vi "jaccard kNN.vi"() -> ()   [LabVIEW 2014]
uses:
  <vilib>/Utility/file.llb/Write To Spreadsheet File (string).vi
panel:
  out "Array 4":string[][](array[string])
  out "Slide 2":dbl(slide) scale=0.0..50.0
  out "Slide":dbl(slide) scale=0.0..9.0
  in  "Path":path
  in  "all rows":string[][](array[string])=array2038x3[6114 elements]
  out "LCS/min (Lsample,Lknown)":dbl[][](array[numeric])
  out "Distance values (LCS)":dbl[][](array[numeric])
  out "size(s)":i32
  out "accuracy":string[][](array[string])
  out "Results":string[][](array[string])
  out "test data (K)":string[][](array[string])
  out "training data (k-1)":string[][](array[string])
  in  "K folds K":i32=10
  out "K folds data":string[][](array[string])
  out "Assigned using LCS (enhanced)":string[][](array[string])
  out "Assigned using LCS":string[][](array[string])
  in  "class labels for training data":string[](array[string])
  in  "kNN k":i32=5
  in  "training data (cluster centers)":string[](array[string])
  in  "test data (patterns in)":string[](array[string])=["0 4 0", "4 0 4", "0 4 0", "4 0 4", "0 4 0", "4 0 4", "0 4 0", "4 0 -2", "0 -2 3", "-2 3 0", "3 0 3", "0 3 0", "3 0 4", "0 4 0", "-2 0 1", "0 1 0", "1 0 -4", "0 -4 4", "-2 2 0", "2 0 -1", "0 -1 -4", "-1 -4 1", "-4 1 0", "1 0 3", "0 3 0", "-1 0 -1", "0 -1 2", "0 -1 1", "-1 1 0", "1 0 4", "0 4 0", "4 0 3", "0 3 -2", "3 -2 0", "-2 0 -2", "0 -2 3", "-2 3 -2", "3 -2 0", "-2 0 4", "0 4 0", "4 0 -2", "0 -2 2", "2 -1 0", "-1 0 4", "0 4 0", "4 0 2", "0 2 0", "2 0 -2", "0 -2 0", "1 -1 0", "-1 0 3", "0 3 0", "3 0 -4", "0 -4 4", "-4 4 -4", "4 -4 0", "2 -1 0", "-1 0 3", "0 3 -2", "3 -2 0", "-2 0 -3", "0 -3 0", "-3 0 3", "0 3 0", "3 0 -3", "0 -3 0", "0 4 0", "4 0 4", "0 4 -4", "4 -4 1", "-4 1 -1", "1 -1 0", "-1 0 -3", "0 -3 0", "-3 0 1", "0 1 -4", "1 -4 1", "-4 1 0", "1 0 4", "0 4 0", "4 0 -4", "0 -4 0", "-4 0 -4", "0 -4 4", "-4 4 -4", "4 -4 1", "0 -4 1", "-4 1 0", "1 0 -4", "0 -4 4", "0 4 0", "4 0 -2", "0 -2 2", "-2 2 -2", "2 -2 2", "-2 2 -2", "2 -2 2", "-2 2 -1", "2 -1 0", "-1 0 4", "0 4 0", "4 0 2", "0 2 0", "2 0 4", "0 4 0", "4 0 2", "0 2 -2", "2 -2 0", "-2 0 4", "1 0 -1", "0 -1 0", "-1 0 -1", "0 -1 0", "-1 0 1", "0 1 -1", "-2 2 -2", "2 -2 3", "1 0 -1", "0 -1 0", "-1 0 -1", "0 -1 2", "-1 2 0", "2 0 2", "0 2 -2", "2 -2 0", "-2 0 -4", "0 -4 0", "-2 2 0", "2 0 3", "0 3 -2", "3 -2 2", "1 -1 0", "-1 0 3", "0 4 0", "-2 0 1", "0 1 -4", "1 -4 0", "-4 0 -3", "0 -3 0", "1 0 -1", "0 -1 2", "-1 2 -1", "2 -1 1", "-1 1 -4", "-2 0 -1", "0 -1 1", "0 3 0", "3 0 3", "0 3 0", "3 0 3", "0 3 -2", "-4 0 -4", "0 -4 4", "0 4 0", "4 0 -4", "0 -4 0", "-4 0 -4", "-2 2 0", "2 0 4", "0 4 -4", "4 -4 0", "-4 0 2", "0 2 -2"]
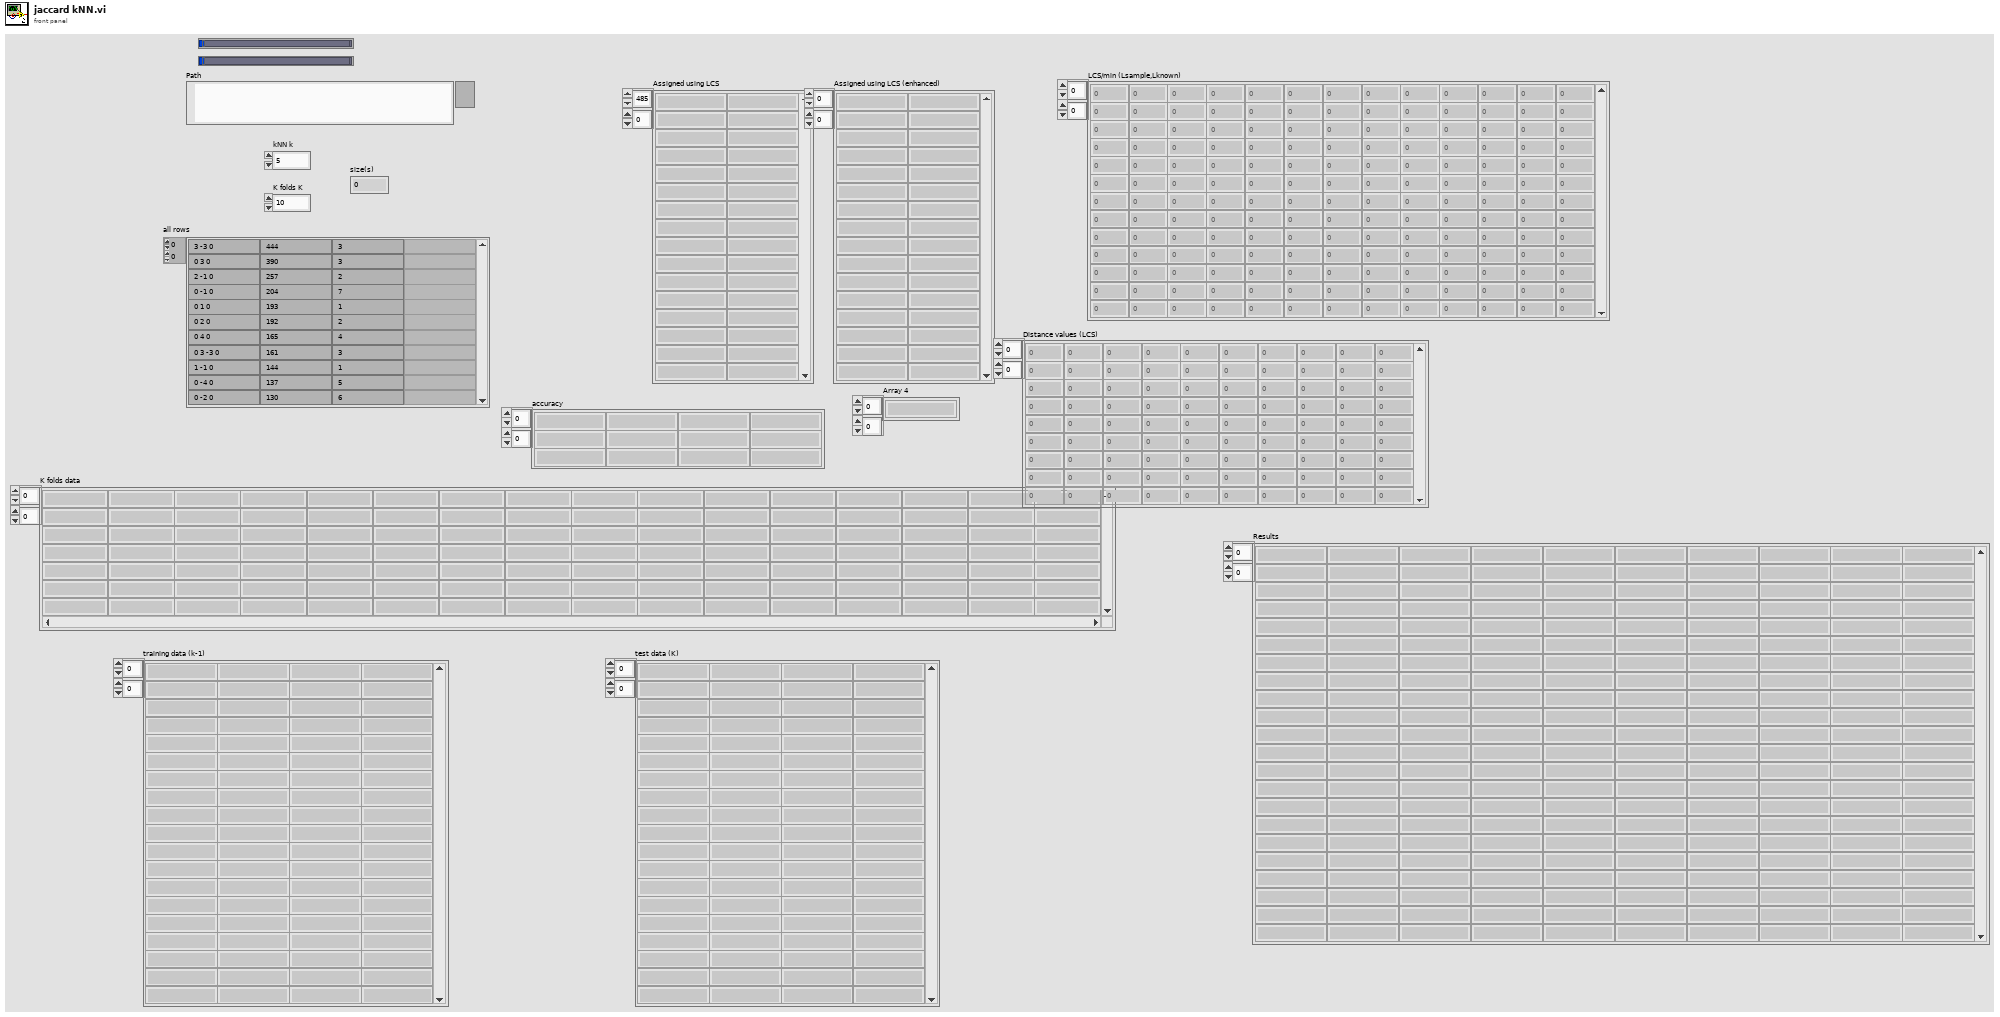
[diagram p1: front panel]
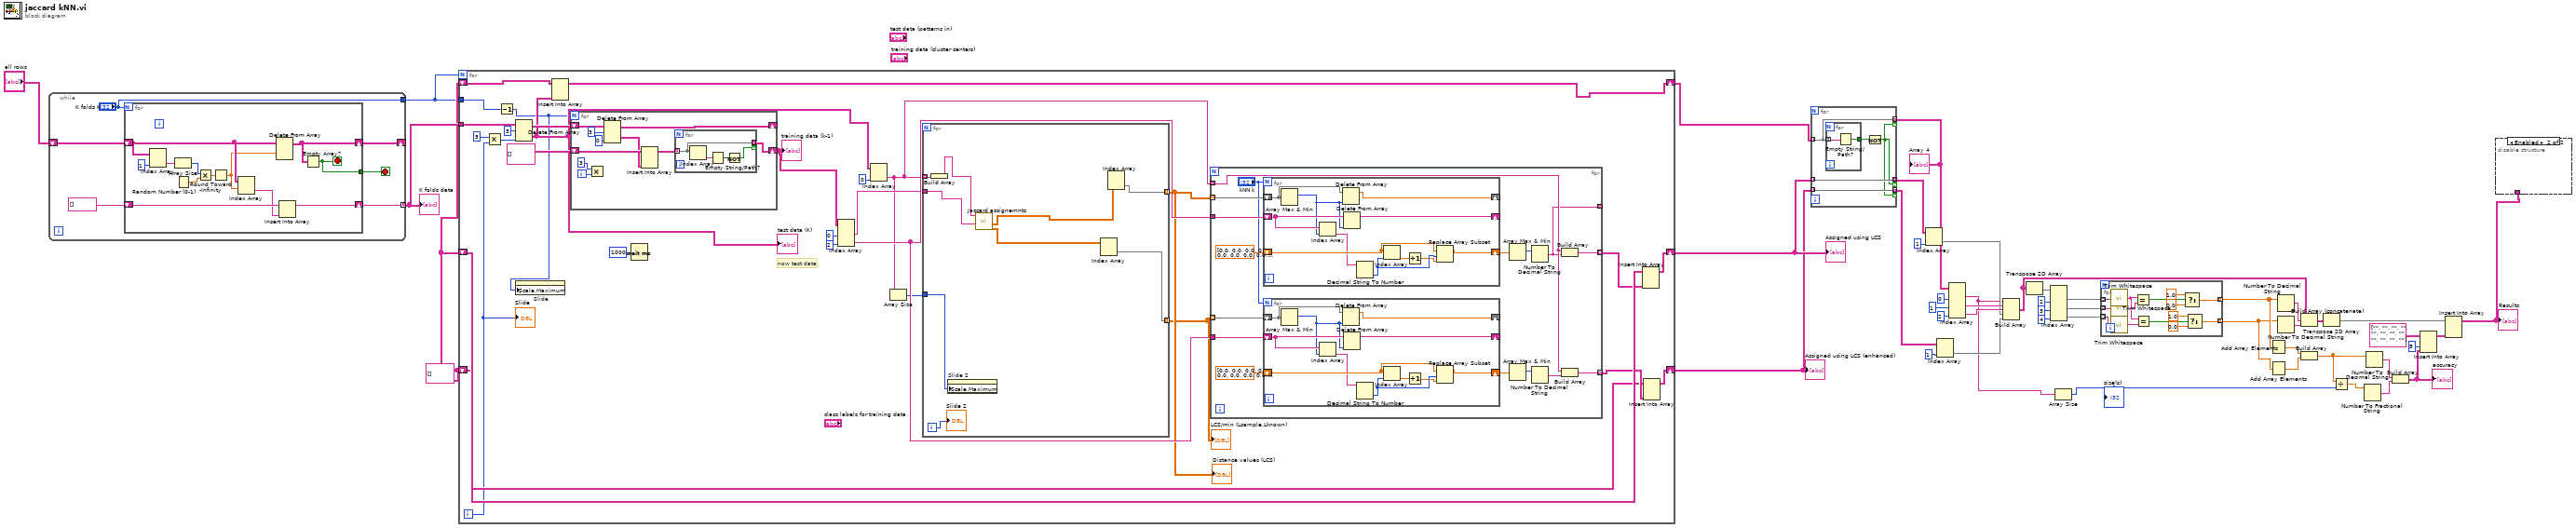
[diagram p0: block diagram]
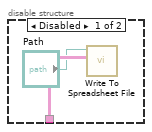
[diagram p2: hidden frame]
diagram:
  w10 = string[][] []
  n1 = while {
    shift-right: [w49] -> _
    shift-left: "all rows" -> [w50]
    tunnel: [w51] -> w46 mode=indexing
    tunnel: ["K folds K"] -> w2
    stop <- w48 stop-if-true
    n2 = for {
      N: "K folds K" -> [_]
      shift-right: [w57] -> w51
      shift-left: string[] [] ("all rows 2") -> [w64]
      shift-right: [w55] -> w49
      shift-left: w50 -> [w56]
      tunnel: [w54] -> w48
      stop <- w54 stop-if-true
      n3 = Index Array(array=w56, index (col)=1 ("disabled index (col)")) -> (element=w60:string[])  [unwired: 1 in]
      n4 = Array Size(array=w60) -> (size(s)=w61:i32)
      n5 = Random Number (0-1)() -> (number: 0 to 1=w62:dbl)
      n6 = Multiply(x=w61, y=w62) -> (x*y=w63:dbl)
      n7 = Round Toward -Infinity(1:w63) -> (0:w53:dbl)
      n8 = Index Array(array=w56, index (row)=w53) -> (element=w58:string[])  [unwired: 1 in]
      n9 = Delete From Array(array=w56, index (row)=w53) -> (array with subset deleted=w55:string[][])  [unwired: 2 in, 1 out]
      n10 = Insert Into Array(array=w64, new element=w58) -> (w57:string[])  [unwired: 1 in]
      n11 = Empty Array?(array=w55) -> (empty?=w54:bool)
    }
  }
  "K folds data" <- w46
  n12 = for {
    N: w2 -> [_]
    tunnel: w46 -> [w93]
    tunnel: w2 -> [w69]
    shift-right: [w76] -> w8
    shift-left: w10 -> [w78]
    shift-right: [w73] -> w7
    shift-left: w10 -> [w75]
    shift-right: [w70] -> w5
    shift-left: w10 -> [w71]
    i -> [w68]
    # "now test data"
    n13 = Multiply(x=3, y=w68) -> (x*y=w82:i32)
    n14 = Decrement(x=w69) -> (x-1=w65:i32)
    n15 = Delete From Array(array=w93, length=3, index (col)=w82) -> (deleted portion=w77:string[][], array with subset deleted=w81:string[][])  [unwired: 1 in]
    "test data (K)" <- w77
    n16 = property on="Slide" class="Slide (strict)"("Scale.Maximum"=w65) -> ()  [unwired: 2 in, 2 out]
    n17 = Insert Into Array(array=w78, new element=w77) -> (w76:string[][])  [unwired: 2 in]
    n18 = for {
      N: w65 -> [_]
      shift-right: [w94] -> w85
      shift-left: string[][] [] ("all rows 2") -> [w102]
      shift-right: [w97] -> _
      shift-left: w81 -> [w103]
      i -> [w99]
      n19 = Multiply(x=3, y=w99) -> ()  [unwired: 1 out]
      n20 = Delete From Array(array=w103, length=3 ("index (col)"), index (col)=0 ("disabled index (col)")) -> (deleted portion=w101:string[][], array with subset deleted=w97:string[][])  [unwired: 1 in]
      n21 = Insert Into Array(array=w102, new element=w101) -> (w95:string[][])  [unwired: 2 in]
      n22 = for {
        tunnel: w95 -> [w106] mode=indexing
        tunnel: [w106] -> w94 mode=indexing if=w107
        n23 = Index Array(array=w106) -> (element=w105:string)  [unwired: 1 in]
        n24 = Empty String/Path?(string/path=w105) -> (empty?=w104:bool)
        n25 = Not(x=w104) -> (.not. x?=w107:bool)
      }
    }
    "training data (k-1)" <- w85
    n26 = Wait (ms)(milliseconds to wait=u32 1000) -> ()  [unwired: 1 out]
    n27 = Index Array(array=w85, index (col) #1=0 ("disabled index (col)"), index (col) #2=2 ("index (col)")) -> (element #1=w88:string[], element #2=w89:string[])  [unwired: 2 in]
    n28 = Index Array(array=w77, index (col)=0 ("disabled index (col)")) -> (element=w67:string[])  [unwired: 1 in]
    n29 = Array Size(array=w67) -> (size(s)=w66:i32)
    n30 = for {
      tunnel: w67 -> [w154] mode=indexing
      tunnel: w88 -> [w150]
      tunnel: [w149] -> w87 mode=indexing
      tunnel: [w148] -> w86 mode=indexing
      tunnel: w66 -> [w152]
      i -> [w153]
      n31 = Build Array(w154) -> (w151:string[])
      n32 = property on="Slide 2" class="Slide (strict)"("Scale.Maximum"=w152) -> ()  [unwired: 2 in, 2 out]
      n33 = call "Jaccard assignemnts.vi"("cluster centers in"=w150, "patterns in"=w151) -> ("distance values out enhanced multiset)"=w147:dbl[][], "distance values out (multiset)"=w146:dbl[][])  [unwired: 6 in, 2 out]
      n34 = Index Array(array=w147) -> (element=w148:dbl[])  [unwired: 2 in]
      n35 = Index Array(array=w146) -> (element=w149:dbl[])  [unwired: 2 in]
      "Slide 2" <- w153
    }
    "Distance values (LCS)" <- w87
    "LCS/min (Lsample,Lknown)" <- w86
    n36 = for {
      tunnel: w67 -> [w114] mode=indexing
      tunnel: w87 -> [w123] mode=indexing
      tunnel: w89 -> [w122]
      tunnel: w86 -> [w113] mode=indexing
      tunnel: w89 -> [w112]
      tunnel: [w111] -> w74 mode=indexing
      tunnel: [w110] -> w72 mode=indexing
      tunnel: [w108] -> _ mode=indexing
      n37 = for {
        N: "kNN k" -> [_]
        shift-right: [w142] -> _
        shift-left: w123 -> [w145]
        shift-right: [w141] -> _
        shift-left: w122 -> [w144]
        shift-right: [w136] -> w119
        shift-left: dbl[] [0.0, 0.0, 0.0, 0.0, 0.0, 0.0, 0.0, 0.0, 0.0, 0.0, 0.0, 0.0] -> [w137]
        n38 = Array Max & Min(array=w145) -> (max index (indices)=w143:i32)  [unwired: 3 out]
        n39 = Index Array(array=w144, index=w143) -> (element=w135:string)
        n40 = Delete From Array(array=w145, index=w143) -> (array with subset deleted=w142:dbl[])  [unwired: 1 in, 1 out]
        n41 = Delete From Array(array=w144, index=w143) -> (array with subset deleted=w141:string[])  [unwired: 1 in, 1 out]
        n42 = Decimal String To Number(string=w135) -> (number=w140:i32)  [unwired: 2 in, 1 out]
        n43 = Index Array(array=w137, index=w140) -> (element=w138:dbl)
        n44 = Increment(x=w138) -> (x+1=w139:dbl)
        n45 = Replace Array Subset(array=w137, new element=w139, index=w140) -> (w136:dbl[])
      }
      n46 = for {
        N: "kNN k" -> [_]
        shift-right: [w131] -> _
        shift-left: w113 -> [w134]
        shift-right: [w130] -> _
        shift-left: w112 -> [w133]
        shift-right: [w125] -> w117
        shift-left: dbl[] [0.0, 0.0, 0.0, 0.0, 0.0, 0.0, 0.0, 0.0, 0.0, 0.0, 0.0, 0.0] -> [w126]
        n47 = Array Max & Min(array=w134) -> (max index (indices)=w132:i32)  [unwired: 3 out]
        n48 = Index Array(array=w133, index=w132) -> (element=w124:string)
        n49 = Delete From Array(array=w134, index=w132) -> (array with subset deleted=w131:dbl[])  [unwired: 1 in, 1 out]
        n50 = Delete From Array(array=w133, index=w132) -> (array with subset deleted=w130:string[])  [unwired: 1 in, 1 out]
        n51 = Decimal String To Number(string=w124) -> (number=w129:i32)  [unwired: 2 in, 1 out]
        n52 = Index Array(array=w126, index=w129) -> (element=w127:dbl)
        n53 = Increment(x=w127) -> (x+1=w128:dbl)
        n54 = Replace Array Subset(array=w126, new element=w128, index=w129) -> (w125:dbl[])
      }
      n55 = Array Max & Min(array=w119) -> (max index (indices)=w120:i32)  [unwired: 3 out]
      n56 = Array Max & Min(array=w117) -> (max index (indices)=w116:i32)  [unwired: 3 out]
      n57 = Number To Decimal String(number=w120) -> (decimal integer string=w108:string)  [unwired: 1 in]
      n58 = Number To Decimal String(number=w116) -> (decimal integer string=w118:string)  [unwired: 1 in]
      n59 = Build Array(w114, w108) -> (w111:string[])
      n60 = Build Array(w114, w118) -> (w110:string[])
    }
    n61 = Insert Into Array(array=w75, new element=w74) -> (w73:string[][])  [unwired: 2 in]
    n62 = Insert Into Array(array=w71, new element=w72) -> (w70:string[][])  [unwired: 2 in]
    "Slide" <- w68
  }
  "Assigned using LCS" <- w7
  "Assigned using LCS (enhanced)" <- w5
  n63 = for {
    tunnel: w8 -> [w158] mode=indexing
    tunnel: [w158] -> w6 mode=indexing if=w155
    tunnel: w7 -> [w157] mode=indexing
    tunnel: [w157] -> w3 mode=indexing if=w155
    tunnel: [w156] -> w4 mode=indexing if=w155
    tunnel: w5 -> [w156] mode=indexing
    n64 = for {
      tunnel: w158 -> [w161] mode=indexing
      tunnel: [w160] -> w159
      n65 = Empty String/Path?(string/path=w161) -> (empty?=w160:bool)
    }
    n66 = Not(x=w159) -> (.not. x?=w155:bool)
  }
  "Array 4" <- w6
  n67 = Index Array(array=w3, index (col)=1 ("disabled index (col)")) -> (element=w16:string[])  [unwired: 1 in]
  n68 = Index Array(array=w4, index (col)=1 ("disabled index (col)")) -> (element=w14:string[])  [unwired: 1 in]
  n69 = Index Array(array=w6, index (col) #1=0 ("disabled index (col)"), index (col) #2=1 ("index (col)"), index (col) #3=2 ("index (col)")) -> (element #1=w12:string[], element #2=w19:string[], element #3=w18:string[])  [unwired: 3 in]
  n70 = Build Array(w12, w19, w18, w16, w14) -> (w13:string[][])
  n71 = Transpose 2D Array(2D array=w13) -> (transposed array=w37:string[][])
  n72 = Index Array(array=w37, index (col) #1=2 ("disabled index (col)"), index (col) #2=3 ("index (col)"), index (col) #3=4 ("index (col)")) -> (element #1=w40:string[], element #2=w39:string[], element #3=w38:string[])  [unwired: 3 in]
  n73 = Array Size(array=w12) -> (size(s)=w11:i32)
  "size(s)" <- w11
  n74 = for {
    tunnel: w40 -> [w167] mode=indexing
    tunnel: w39 -> [w166] mode=indexing
    tunnel: w38 -> [w165] mode=indexing
    tunnel: [w169] -> w22 mode=indexing
    tunnel: [w168] -> w21 mode=indexing
    n75 = call <vilib>:"Trim Whitespace.vi"("string"=w166) -> ("trimmed string"=w164:string)  [unwired: 1 in]
    n76 = call <vilib>:"Trim Whitespace.vi"("string"=w165) -> ("trimmed string"=w163:string)  [unwired: 1 in]
    n77 = call <vilib>:"Trim Whitespace.vi"("string"=w167) -> ("trimmed string"=w162:string)  [unwired: 1 in]
    n78 = Equal?(x=w162, y=w164) -> (x = y?=w175:bool)
    n79 = Equal?(x=w162, y=w163) -> (x = y?=w170:bool)
    n80 = Select(t=1.0, s=w175, f=0.0) -> (s? t:f=w169:dbl)
    n81 = Select(t=1.0, s=w170, f=0.0) -> (s? t:f=w168:dbl)
  }
  n82 = Add Array Elements(numeric array=w22) -> (sum=w23:dbl)
  n83 = Add Array Elements(numeric array=w21) -> (sum=w24:dbl)
  n84 = Number To Decimal String(number=w22) -> (decimal integer string=w36:string[])  [unwired: 1 in]
  n85 = Number To Decimal String(number=w21) -> (decimal integer string=w35:string[])  [unwired: 1 in]
  n86 = Build Array (concatenate)(w13, w36, w35) -> (w34:string[][])
  n87 = Build Array(w23, w24) -> (w25:dbl[])
  n88 = Transpose 2D Array(2D array=w34) -> (transposed array=w20:string[][])
  n89 = Divide(x=w25, y=w11) -> (x/y=w26:dbl[])
  n90 = Number To Fractional String(number=w26) -> (F-format string=w28:string[])  [unwired: 3 in]
  n91 = Number To Decimal String(number=w25) -> (decimal integer string=w27:string[])  [unwired: 1 in]
  n92 = Build Array(w27, w28) -> (w32:string[][])
  "accuracy" <- w32
  n93 = Insert Into Array(array=string[][] [["", "", "", "", "", ""], ["", "", "", "", "", ""]] ("appended array 3"), index (col)=5 ("disabled index (col)"), new element=w32) -> (w31:string[][])  [unwired: 1 in]
  n94 = Insert Into Array(array=w20, new element=w31) -> (w9:string[][])  [unwired: 2 in]
  "Results" <- w9
  n95 = disable-structure shown="Enabled" {
    disable-tunnel: w9 -> [w177 _]
    frame Disabled {
      n96 = call-poly <vilib>:"Write To Spreadsheet File.vi"("2D data"=w177, "file path (dialog if empty)"="Path") -> ()  [unwired: 6 in, 1 out]
    }
    frame Enabled {
    }
  }
